vi "GetSetProfileInfo.vi"(4 "Parameter":enum16{"Logo Path", "Logo", "Title", "Rounds"}(ring), 6 "Get/Set State":enum16{"Get", "Set", "Load"}(ring), 8 "Rounds To Show In":i32, 9 "Logo Path In":path, 10 "Title":string, 11 "image data":T1) -> (0 "Rounds To Show Out":i32, 1 "Logo Path Out":path, 2 "Title":string, 3 "image data out":T1)   [LabVIEW 2013]
uses:
  <vilib>/picture/picture.llb/imagedata.ctl
  <vilib>/Utility/sysdir.llb/System Directory Type.ctl
  <vilib>/Utility/xml.llb/Read From XML File(string).vi
  <vilib>/Utility/xml.llb/Write to XML File(string).vi
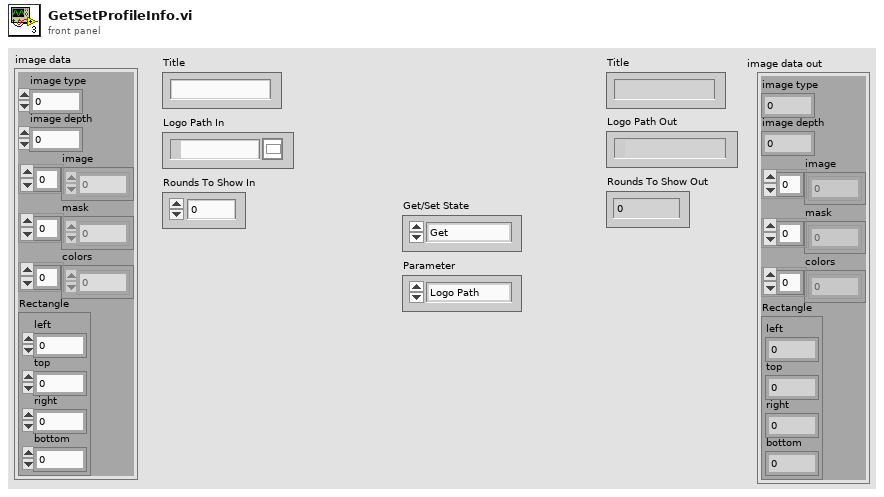
[diagram p1: front panel]
types:
  T1 = typedef "imagedata.ctl" = cluster{"image type":i32, "image depth":i32, "image":u8[], "mask":u8[], "colors":u32[], "Rectangle":cluster{"left":i16, "top":i16, "right":i16, "bottom":i16}}
  T2 = typedef "System Directory Type.ctl" = i32
  T3 = cluster{"Logo Path In":path, "Title":string, "image data":T1, "Rounds To Show In":i32}
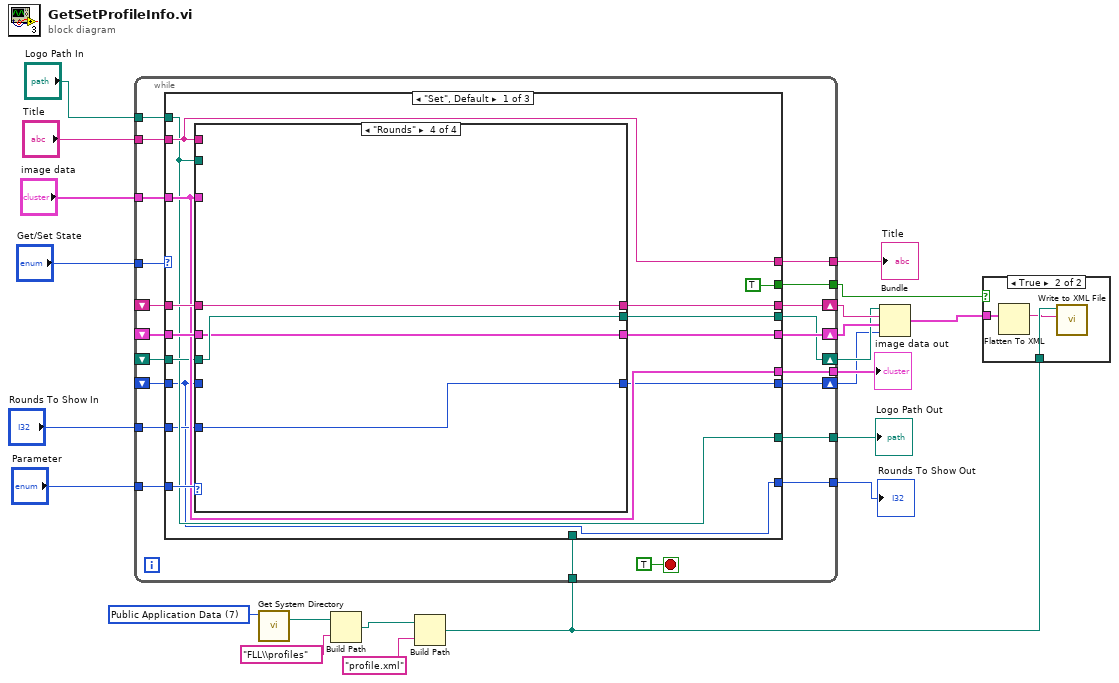
[diagram p0: block diagram]
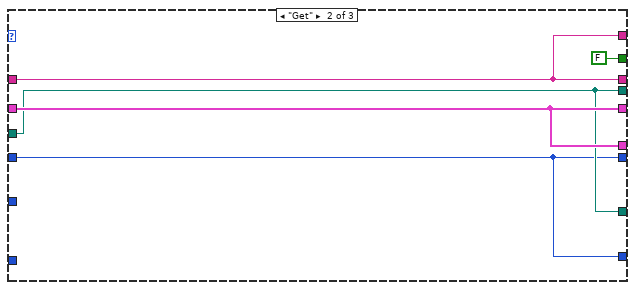
[diagram p6: hidden frame]
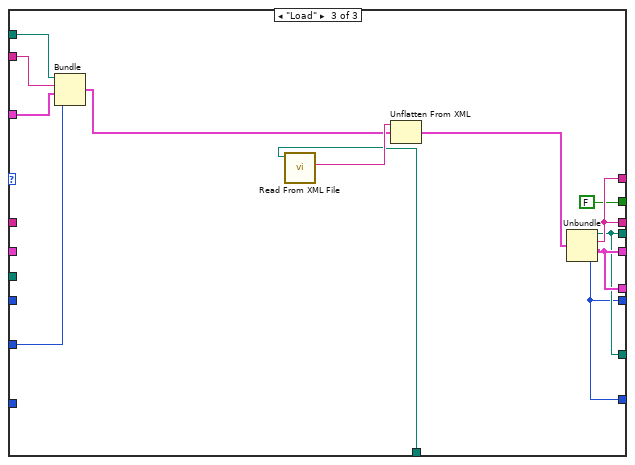
[diagram p7: hidden frame]
diagram:
  w10 = T2 7 items=["User Home"=0, "User Desktop"=1, "User Documents"=2, "User Application Data"=3, "User Preferences"=4, "User Temporary"=5, "Public Documents"=6, "Public Application Data"=7, "Public Preferences"=8, "Public Cache"=13, "System Core Libraries"=9, "System Installed Libraries"=10, "Application Files"=11, "Boot Volume Root"=12] ("system directory type")
  n1 = call <vilib>:"Get System Directory.vi"("system directory type"=w10) -> ("system directory"=w12:path)  [unwired: 10 in]
  n2 = Build Path(base path=w12, name or relative path="FLL\\profiles") -> (appended path=w13:path)
  n3 = Build Path(base path=w13, name or relative path="profile.xml") -> (appended path=w8:path)
  n4 = while {
    shift-right: [w35] -> w16
    shift-left: _ -> [w40]
    shift-right: [w36] -> w15
    shift-left: _ -> [w39]
    tunnel: "Get/Set State" -> [w42]
    tunnel: "Parameter" -> [w41]
    tunnel: "Title" -> [w38]
    tunnel: "image data" -> [w37]
    tunnel: [w34] -> w18
    tunnel: [w33] -> w17
    tunnel: w8 -> [w32]
    shift-right: [w30] -> w5
    shift-left: _ -> [w28]
    tunnel: "Logo Path In" -> [w31]
    tunnel: [w29] -> w6
    tunnel: [w27] -> w4
    shift-right: [w24] -> w1
    shift-left: _ -> [w25]
    tunnel: "Rounds To Show In" -> [w26]
    tunnel: [w23] -> w2
    stop <- TRUE stop-if-true
    n5 = case shown="\"Set\", Default" w42 {
      tunnel: w41 -> [w57 _ _]
      tunnel: w40 -> [w56 w77 _]
      tunnel: w39 -> [w55 w76 _]
      tunnel: w38 -> [w52 _ w90]
      tunnel: w37 -> [w51 _ w89]
      tunnel: [w54 w76 w84] -> w36
      tunnel: [w53 w77 w83] -> w35
      tunnel: [w51 w76 w84] -> w34
      tunnel: [w52 w77 w83] -> w33
      tunnel: w32 -> [_ _ w86]
      tunnel: w31 -> [w48 _ w85]
      tunnel: [w50 w75 w82] -> w30
      tunnel: [w48 w75 w82] -> w29
      tunnel: w28 -> [w49 w75 _]
      tunnel: [TRUE FALSE FALSE] -> w27
      tunnel: w26 -> [w45 _ w80]
      tunnel: w25 -> [w44 w74 _]
      tunnel: [w46 w74 w79] -> w24
      tunnel: [w44 w74 w79] -> w23
      frame "Set", Default {
        n6 = case shown="\"Rounds\"" w57 {
          tunnel: w56 -> [_ w64 w69 w70]
          tunnel: w55 -> [w60 _ w68 w71]
          tunnel: w52 -> [w61 _ _ _]
          tunnel: w51 -> [_ w65 _ _]
          tunnel: [w60 w65 w68 w71] -> w54
          tunnel: [w61 w64 w69 w70] -> w53
          tunnel: w49 -> [w59 w63 _ w72]
          tunnel: [w59 w63 w67 w72] -> w50
          tunnel: w48 -> [_ _ w67 _]
          tunnel: w44 -> [w58 w62 w66 _]
          tunnel: [w58 w62 w66 w73] -> w46
          tunnel: w45 -> [_ _ _ w73]
          frame "Title", Default {
          }
          frame "Logo" {
          }
          frame "Logo Path" {
          }
          frame "Rounds" {
          }
        }
      }
      frame "Get" {
      }
      frame "Load" {
        n7 = Bundle("Logo Path In"=w85, "Title"=w90, "image data"=w89, "Rounds To Show In"=w80) -> (w88:T3)  [unwired: 1 in]
        n8 = call-poly <vilib>:"Read From XML File.vi"("XML File Path"=w86) -> ("XML Elements"=w91:string)  [unwired: 8 in, 2 out]
        n9 = Unflatten From XML(xml string=w91, type=w88) -> (value=w87:T3)  [unwired: 1 in, 1 out]
        n10 = Unbundle(w87) -> ("Logo Path In"=w82:path, "Title"=w83:string, "image data"=w84:T1, "Rounds To Show In"=w79:i32)
      }
    }
  }
  "Title" <- w17
  "image data out" <- w18
  "Logo Path Out" <- w6
  "Rounds To Show Out" <- w2
  n11 = Bundle("Logo Path In"=w5, "Title"=w16, "image data"=w15, "Rounds To Show In"=w1) -> (w9:T3)  [unwired: 1 in]
  n12 = case shown="True" w4 {
    tunnel: w9 -> [_ w94]
    tunnel: w8 -> [_ w93]
    frame False {
    }
    frame True {
      n13 = Flatten To XML(anything=w94) -> (xml string=w92:string)
      n14 = call-poly <vilib>:"Write to XML File.vi"("XML Input"=w92, "XML File Path"=w93) -> ()  [unwired: 7 in, 3 out]
    }
  }
